vi "GetPort.vi"(8 "error in (no error)":errorcluster, 10 "Port":u8, 11 "Cypress CY8CKIT-059 in":refnum<class "Cypress CY8CKIT-059.lvclass">) -> (0 "error out":errorcluster, 1 "Response":string, 2 "Value":u8, 3 "Cypress CY8CKIT-059 out":refnum<class "Cypress CY8CKIT-059.lvclass">)   [LabVIEW 2020, in "Cypress CY8CKIT-059.lvclass"]
doc: "Get the status of a digital port on the target device."
uses:
  Cypress CY8CKIT-059.lvclass
  Controls/Device Code.ctl
  Controls/Device Command Code.ctl
  Cypress CY8CKIT-059.lvclass/Cypress CY8CKIT-059.ctl
  956829cf-2784-4d14-9b05-d593b18957b2.vi
  Read Serial Port.vi
  Write Serial Port.vi
  <vilib>/Utility/error.llb/Error Cluster From Error Code.vi
  <vilib>/ErrorRing/Error Ring.xnode
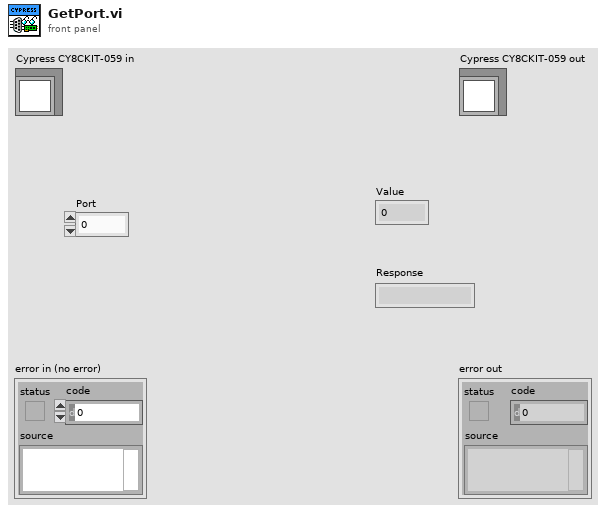
[diagram p1: front panel]
types:
  T1 = typedef "Device Command Code.ctl" = string
  T2 = typedef "Device Code.ctl" = string
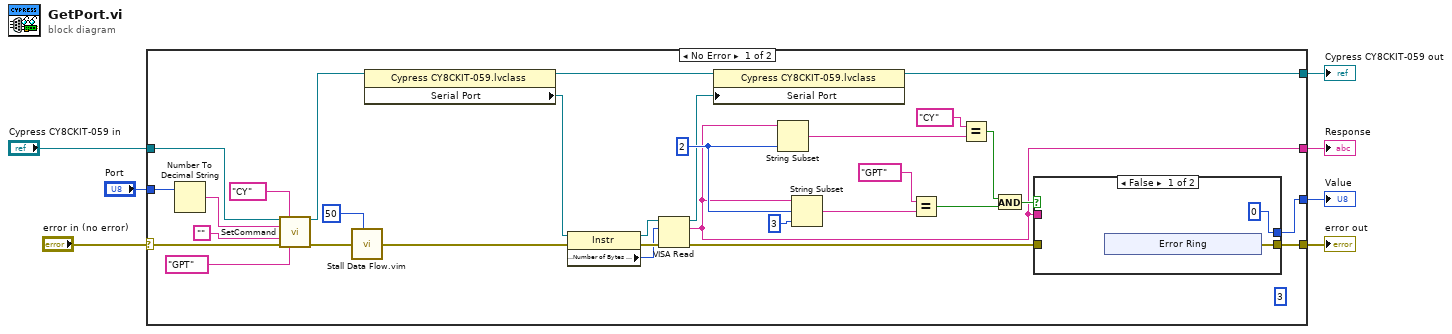
[diagram p0: block diagram]
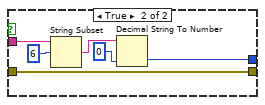
[diagram p2: hidden frame]
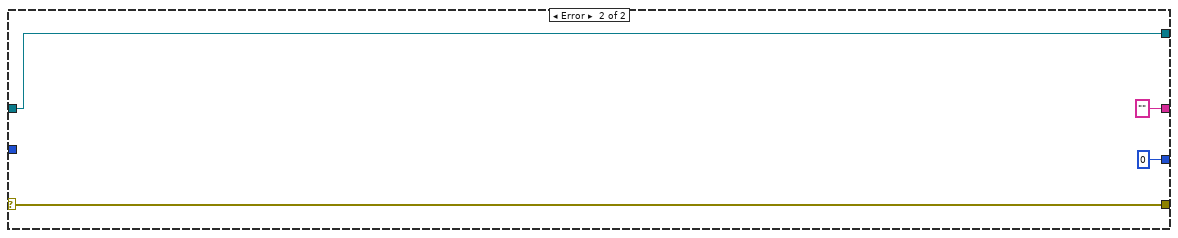
[diagram p3: hidden frame]
diagram:
  n1 = case shown="No Error" "error in (no error)" {
    selector: "error in (no error)" -> [w38 w54]
    tunnel: [w19 w54] -> w3
    tunnel: "Cypress CY8CKIT-059 in" -> [w36 w55]
    tunnel: [w15 w55] -> w2
    tunnel: "Port" -> [w34 _]
    tunnel: [w9 "" ("read buffer")] -> w4
    tunnel: [w8 u8 0] -> w1
    frame No Error {
      (unwired) 3 ("length (rest)")
      w25 = 2 ("length (rest)")
      n2 = Number To Decimal String(number=w34) -> (decimal integer string=w33:string)  [unwired: 1 in]
      n3 = call-dynamic "SetCommand.vi"("Cypress CY8CKIT-059 in"=w36, "Device Code"=T2 "CY", "Parameter 1"=w33, "Parameter 3"="", "error in (no error)"=w38, "Command Code"=T1 "GPT") -> ("Cypress CY8CKIT-059 out"=w31:refnum<class "Cypress CY8CKIT-059.lvclass">, "error out"=w12:errorcluster)  [unwired: 7 in, 1 out]
      n4 = call "Stall Data Flow.vim"("value in"=w12, "milliseconds to wait"=u32 50) -> ("value out"=w11:errorcluster)  [unwired: 1 out]
      n5 = property class="Cypress CY8CKIT-059.lvclass"(reference=w31) -> (reference out=w16:refnum<class "Cypress CY8CKIT-059.lvclass">, "Serial Port"=w30:refnum<visa-resource-name>)  [unwired: 1 in, 1 out]
      n6 = property class="Instr"(reference=w30, error in=w11) -> (reference out=w28:refnum<visa-resource-name>, error out=w29:errorcluster, "Serial Settings:Number of Bytes at Serial Port"=w27:u32)
      n7 = VISA Read(VISA resource name=w28, byte count=w27, error in (no error)=w29) -> (VISA resource name out=w14:refnum<visa-resource-name>, read buffer=w9:string, error out=w20:errorcluster)  [unwired: 1 out]
      n8 = property class="Cypress CY8CKIT-059.lvclass"(reference=w16, "Serial Port"=w14) -> (reference out=w15:refnum<class "Cypress CY8CKIT-059.lvclass">)  [unwired: 1 in, 1 out]
      n9 = String Subset(string=w9, length (rest)=w25) -> (substring=w17:string)  [unwired: 1 in]
      n10 = String Subset(string=w9, offset (0)=w25, length (rest)=3 ("length (rest)")) -> (substring=w26:string)
      n11 = Equal?(x=T1 "GPT" ("Command Code"), y=w26) -> (x = y?=w22:bool)
      n12 = Equal?(x=T2 "CY" ("Device Code"), y=w17) -> (x = y?=w18:bool)
      n13 = And(x=w18, y=w22) -> (x .and. y?=w21:bool)
      n14 = case shown="False" w21 {
        tunnel: w20 -> [_ w51]
        tunnel: [w40 w51] -> w19
        tunnel: w9 -> [_ w50]
        tunnel: [u8 0 w46] -> w8
        frame False {
          n15 = xnode "Error Ring"() -> ("error out"=w40:errorcluster)
        }
        frame True {
          n16 = String Subset(string=w50, offset (0)=6) -> (substring=w48:string)  [unwired: 1 in]
          n17 = Decimal String To Number(string=w48, default (0L)=u8 0 ("default (0 I32)")) -> (number=w46:u8)  [unwired: 1 in, 1 out]
        }
      }
    }
    frame Error {
    }
  }
  "error out" <- w3
  "Cypress CY8CKIT-059 out" <- w2
  "Response" <- w4
  "Value" <- w1
